vi "Simulation.vi"(8 "error in (no error)":errorcluster, 11 "MB Sim Base in":refnum<class "MB Slave Simulator Base.lvclass">) -> (0 "error out":errorcluster)   [LabVIEW 2021, in "MB Slave Simulator Base.lvclass"]
uses:
  MB Slave Simulator Base.lvclass
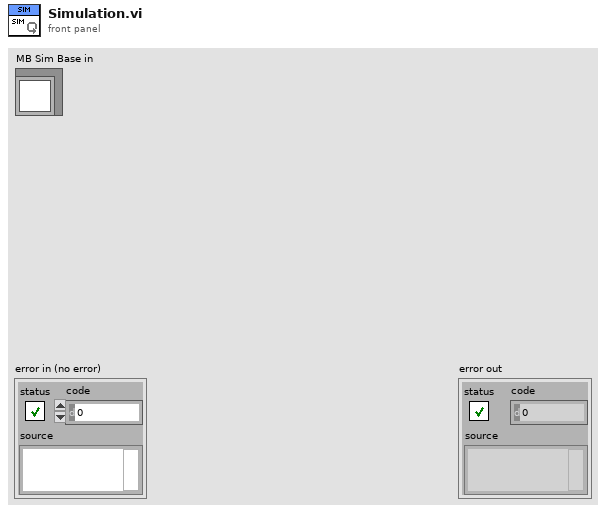
[diagram p1: front panel]
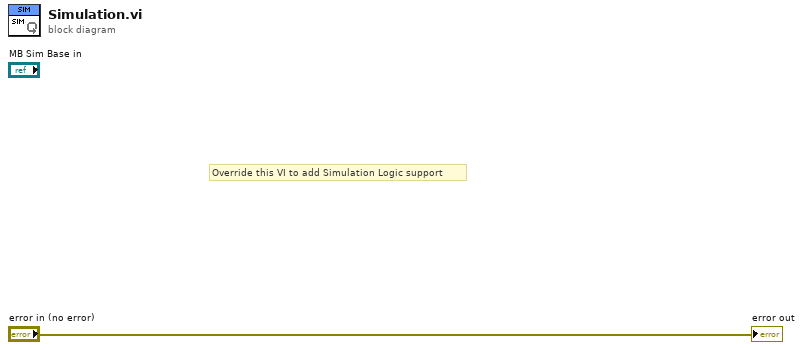
[diagram p0: block diagram]
diagram:
  # "Override this VI to add Simulation Logic support"
  "error out" <- "error in (no error)"
